vi "Unregister.vi"(8 "error in (no error)":errorcluster, 9 "Time out (1000 ms)":i32=1000, 10 "URI":string, 11 "WAMP Client in":refnum<class "WAMP Client.lvclass">) -> (0 "error out":errorcluster, 1 "WAMP Error":T1={"Details"="{}", "ArgumentKw Payload"="{}", "Error?"=FALSE, "Error URI"="", "Arguments Payload"=""}, 3 "WAMP Client out":refnum<class "WAMP Client.lvclass">)   [LabVIEW 2020, in "wamplv.lvlib" / "WAMP Client.lvclass"]
uses:
  WAMP Client.lvclass
  TypeDefs/WAMP error.ctl
  621c6210-80ea-441c-aa52-19dc047a6863.vi
  <vilib>/Utility/error.llb/Error Cluster From Error Code.vi
  WAMP Client.lvclass/WAMP Client.ctl
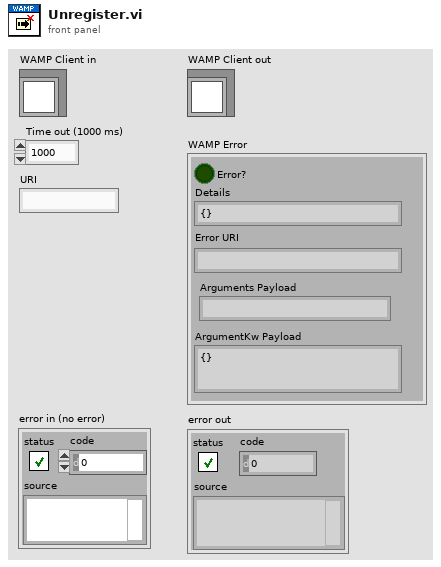
[diagram p1: front panel]
types:
  T1 = typedef "wamplv.lvlib/WAMP Client.lvclass/WAMP error.ctl" = cluster{"Details":string, "ArgumentKw Payload":string, "Error?":bool, "Error URI":string, "Arguments Payload":string}
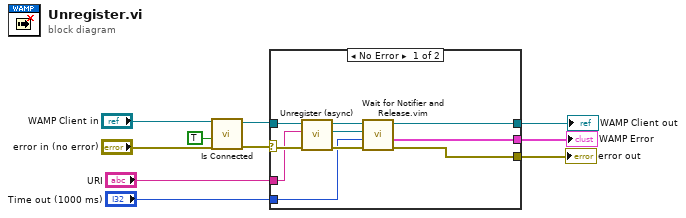
[diagram p0: block diagram]
diagram:
  n1 = call "Is Connected.vi"("error in"="error in (no error)", "Raise error if not connected"=TRUE, "WAMP Client in"="WAMP Client in") -> ("error out"=w5:errorcluster, "WAMP Client out"=w4:refnum<class "WAMP Client.lvclass">)  [unwired: 6 in, 1 out]
  n2 = case shown="No Error" w5 {
    selector: w5 -> [w20 w22]
    tunnel: [w15 w22] -> w10
    tunnel: [w11 w21] -> w9
    tunnel: w4 -> [w19 w21]
    tunnel: "Time out (1000 ms)" -> [w16 _]
    tunnel: "URI" -> [w18 _]
    tunnel: [w14 _] -> w6
    frame No Error {
      n3 = call-dynamic "Unregister (async).vi"("error in (no error)"=w20, "Endpoint URI"=w18, "WAMP Client in"=w19) -> ("error out"=w17:errorcluster, "notifier out"=w12:refnum<notifier>, "WAMP Client out"=w13:refnum<class "WAMP Client.lvclass">)  [unwired: 6 in]
      n4 = call "Wait for Notifier and Release.vim"("error in (no error)"=w17, "timeout in ms (-1)"=w16, "Notifier in"=w12, "WAMP Client in"=w13) -> ("error out"=w15:errorcluster, "WAMP Error"=w14:T1, "WAMP Client out"=w11:refnum<class "WAMP Client.lvclass">)  [unwired: 4 in, 1 out]
    }
    frame Error {
    }
  }
  "error out" <- w10
  "WAMP Client out" <- w9
  "WAMP Error" <- w6
